vi "Keithley 2200 Series Save Instrument Settings.vi"() -> ()   [LabVIEW 2021]
doc: "DESCRIPTION:\n\nThis VI configures the power supply to generate a DC voltage at the output with Over Voltage Protection.\n\nINSTRUCTIONS:\n1. Enter the resource name.\n2. Enter voltage,OVP limit.\n3. Select Save or Recall operation ,to save or recall instrument settings to or from memory \n4. Enter Non -volatile memory address, that the settings will be saved to. \n5. Run the VI.\n\nNOTES:\n\nNotice the order of the power supply component VIs in the block diagram. The first VI in a sequence is the power supply Initialize.vi, which provides a VISA session to the instrument driver. The last VI in a sequence must be the power supply Close.vi which closes the Visa session."
uses:
  <instrlib>/Keithley 2200 Series/Keithley 2200 Series.lvlib
panel:
  in  "Voltage Unit(V)":u16(ring) items=["V", "mV", "kV"]
  in  "Unit(V)":u16(ring) items=["V", "mV", "kV", "A", "mA"]
  in  "Action(0:Save)":u16(ring) items=["Save", "Recall"]
  in  "Memory Address(1)":dbl=1.0
  in  "Manual Range(0.00)":dbl format="%.2f"
  in  "Voltage Limit(0.0V)":dbl format="%_2g"
  in  "VISA resource name":refnum<visa-resource-name>
  # "(c) Copyright 2012 Keithley Instruments Inc  ALL RIGHTS RESERVED."
  # "Over Voltage Protection"
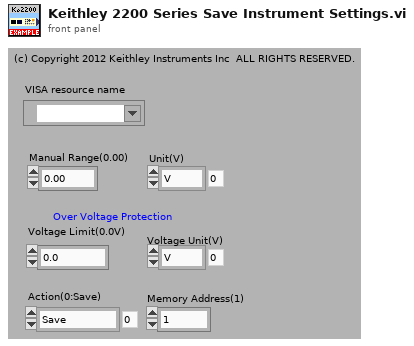
[diagram p1: front panel]
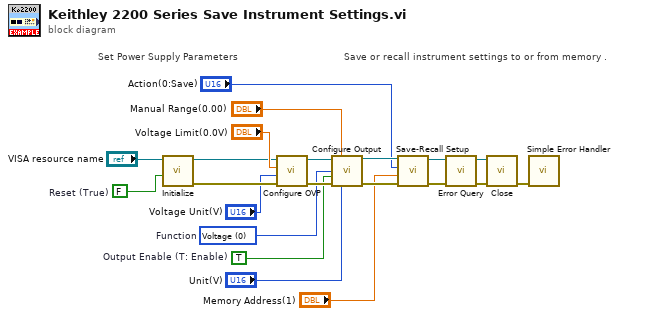
[diagram p0: block diagram]
diagram:
  w7 = FALSE items=["OFF", "ON", "OFF", "ON"]  # Reset (True)
  w11 = u16 0 items=["Voltage", "Current"]  # Function
  w10 = TRUE items=["OFF", "ON", "OFF", "ON"]  # Output Enable (T: Enable)
  # "Set Power Supply Parameters"
  # "Save or recall instrument settings to or from memory ."
  n1 = call <instrlib>:"Initialize.vi"("Reset (True)"=w7, "VISA resource name"="VISA resource name") -> ("error out"=w4:errorcluster, "VISA resource name out"=w5:refnum<visa-resource-name>)  [unwired: 4 in, 4 out]
  n2 = call <instrlib>:"Configure OVP.vi"("error in (no error)"=w4, "Voltage Unit(V)"="Voltage Unit(V)", "Voltage Limit(0.0V)"="Voltage Limit(0.0V)", "VISA resource name"=w5) -> ("error out"=w16:errorcluster, "VISA resource name out"=w17:refnum<visa-resource-name>)  [unwired: 1 in, 5 out]
  n3 = call <instrlib>:"Configure Output.vi"("VISA resource name"=w17, "Manual Range(0.00)"="Manual Range(0.00)", "Function(0:Voltage)"=w11, "Enable Output (T: Enable)"=w10, "error in (no error)"=w16, "Unit(V)"="Unit(V)") -> ("VISA resource name out"=w15:refnum<visa-resource-name>, "error out"=w14:errorcluster)  [unwired: 8 out]
  n4 = call <instrlib>:"Save-Recall Setup.vi"("error in (no error)"=w14, "Memory Address(1)"="Memory Address(1)", "Action(0:Save)"="Action(0:Save)", "VISA resource name"=w15) -> ("error out"=w12:errorcluster, "VISA resource name out"=w13:refnum<visa-resource-name>)  [unwired: 1 in, 5 out]
  n5 = call <instrlib>:"Error Query.vi"("error in (no error)"=w12, "VISA resource name"=w13) -> ("error out"=w20:errorcluster, "VISA resource name out"=w21:refnum<visa-resource-name>)  [unwired: 8 out]
  n6 = call <instrlib>:"Close.vi"("error in (no error)"=w20, "VISA resource name"=w21) -> ("error out"=w18:errorcluster)  [unwired: 9 out]
  n7 = call <vilib>:"Simple Error Handler.vi"("error in (no error)"=w18) -> ()  [unwired: 1 in, 8 out]
